vi "Convert Ohms to Num.vi"(1 "Numeric":dbl) -> (0 "String":string)   [LabVIEW 2013]
panel:
  out "Numeric (SI Notation)":dbl format="%#_6p"
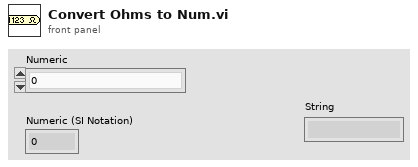
[diagram p1: front panel]
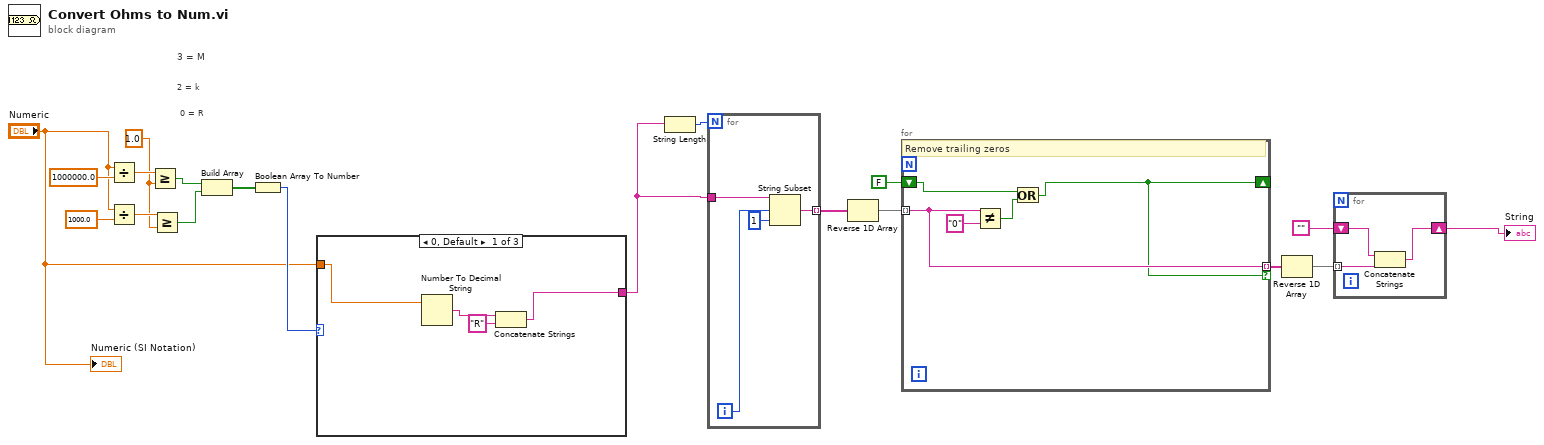
[diagram p0: block diagram]
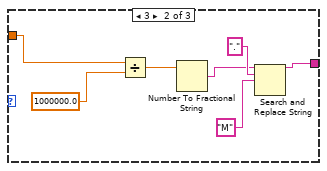
[diagram p2: hidden frame]
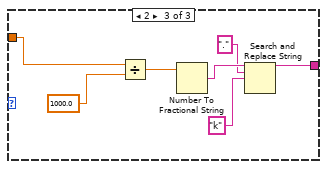
[diagram p3: hidden frame]
diagram:
  w14 = 1.0 ("y")
  # "0 = R"
  # "2 = k"
  # "3 = M"
  n1 = Divide(x="Numeric", y=1000000.0) -> (x/y=w15:dbl)
  n2 = Divide(x="Numeric", y=1000.0) -> (x/y=w16:dbl)
  n3 = Greater Or Equal?(x=w15, y=w14) -> (x >= y?=w13:bool)
  n4 = Greater Or Equal?(x=w16, y=w14) -> (x >= y?=w12:bool)
  n5 = Build Array(w13, w12) -> (w17:bool[])
  n6 = Boolean Array To Number(Boolean array=w17) -> (number=w11:u32)
  n7 = case shown="0, Default" w11 {
    tunnel: "Numeric" -> [w23 w30 w37]
    tunnel: [w20 w24 w31] -> w8
    frame 0, Default {
      n8 = Number To Decimal String(number=w23) -> (decimal integer string=w22:string)  [unwired: 1 in]
      n9 = Concatenate Strings(w22, "R" ("string")) -> (w20:string)
    }
    frame 3 {
      n10 = Divide(x=w30, y=1000000.0) -> (x/y=w28:dbl)
      n11 = Number To Fractional String(number=w28) -> (F-format string=w25:string)  [unwired: 3 in]
      n12 = Search and Replace String(input string=w25, search string=".", replace string="M" ("replace string (\"\")")) -> (result string=w24:string)  [unwired: 5 in, 3 out]
    }
    frame 2 {
      n13 = Divide(x=w37, y=1000.0) -> (x/y=w35:dbl)
      n14 = Number To Fractional String(number=w35) -> (F-format string=w34:string)  [unwired: 3 in]
      n15 = Search and Replace String(input string=w34, search string=".", replace string="k" ("replace string (\"\")")) -> (result string=w31:string)  [unwired: 5 in, 3 out]
    }
  }
  n16 = String Length(string=w8) -> (length=w9:i32)
  n17 = for {
    N: w9 -> [_]
    tunnel: w8 -> [w41]
    tunnel: [w38] -> w7 mode=indexing
    i -> [w40]
    n18 = String Subset(string=w41, offset (0)=w40, length (rest)=1 ("length (rest)")) -> (substring=w38:string)
  }
  n19 = Reverse 1D Array(array=w7) -> (reversed array=w6:string[])
  n20 = for {
    tunnel: w6 -> [w43] mode=indexing
    shift-right: [w42] -> _
    shift-left: FALSE -> [w44]
    tunnel: [w43] -> w4 mode=indexing if=w42
    # "Remove trailing zeros"
    n21 = Not Equal?(x=w43, y="0") -> (x != y?=w45:bool)
    n22 = Or(x=w44, y=w45) -> (x .or. y?=w42:bool)
  }
  n23 = Reverse 1D Array(array=w4) -> (reversed array=w3:string[])
  n24 = for {
    tunnel: w3 -> [w49] mode=indexing
    shift-right: [w47] -> w1
    shift-left: "" -> [w48]
    n25 = Concatenate Strings(w48, w49) -> (w47:string)
  }
  "String" <- w1
  "Numeric (SI Notation)" <- "Numeric"
